vi "List_Active_Events.vi"(2 "Alias Table":string[][](array[string]), 3 "Current Event":cluster{string, string[], dbl[], dbl}, 4 "Update Functions In":cluster{string, string[], dbl[], dbl}[](array[cluster])) -> (0 "Item List":string[](array[string]), 1 "Update Functions Out":cluster{string, string[], dbl[], dbl}[](array[cluster]))   [LabVIEW 2011]
doc: "This VI lists the last event exectued along with all currently updating events, and formats them into an \"Item List\" which can be displayed to the growth sequence operator in Run_Sequence.vi"
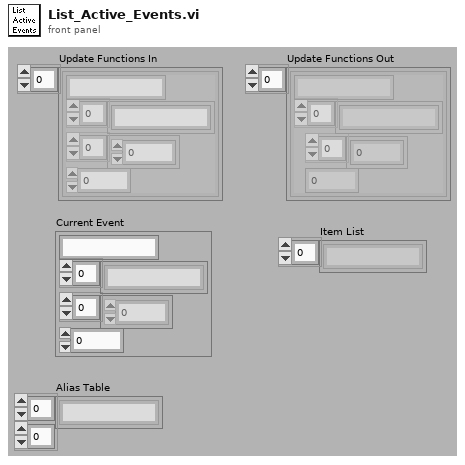
[diagram p1: front panel]
types:
  T1 = enum16{"Discrete", "Continuous", "Instantaneous", "Finite"}
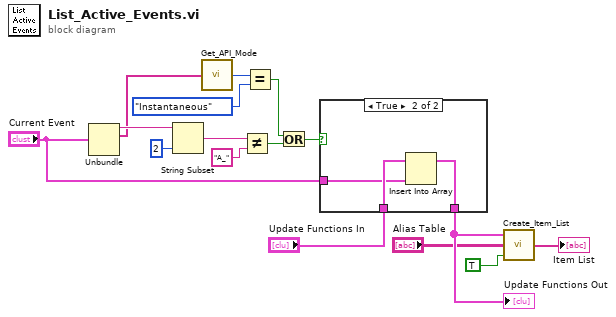
[diagram p0: block diagram]
diagram:
  n1 = Unbundle("Current Event") -> (w14:string, w3:string[])  [unwired: 2 out]
  n2 = String Subset(string=w14, length (rest)=2 ("length (rest)")) -> (substring=w13:string)  [unwired: 1 out]
  n3 = call "Get_API_Mode.vi"("Argument List"=w3) -> ("API Mode"=w6:T1)
  n4 = Not Equal?(x=w13, y="A_") -> (x != y?=w5:bool)
  n5 = Equal?(x=w6, y=T1."Instantaneous" ("API Mode")) -> (x = y?=w4:bool)
  n6 = Or(x=w4, y=w5) -> (x .or. y?=w2:bool)
  n7 = case shown="True" w2 {
    tunnel: "Update Functions In" -> [w17 w20]
    tunnel: [w17 w19] -> w10
    tunnel: "Current Event" -> [_ w18]
    frame False {
    }
    frame True {
      n8 = Insert Into Array(array=w20, new element=w18) -> (w19:cluster{string, string[], dbl[], dbl}[])  [unwired: 1 in]
    }
  }
  "Update Functions Out" <- w10
  n9 = call "Create_Item_List.vi"("Running"=TRUE, "Alias Table"="Alias Table", "Sequence"=w10) -> ("Item List"=→"Item List":string[])
